vi "1_test_1.vi"() -> ()   [LabVIEW 2020]
uses:
  <vilib>/Utility/file.llb/Write Delimited Spreadsheet (DBL).vi
  <vilib>/regexp/Match Regular Expression.xnode
panel:
  out "类型":string
  out "倒数第二步骤 2":string
  out "倒数第三步骤":string
  out "文档名称":string
  out "当前路径文件为：":string
  in  "数字":dbl
  in  "字符串 3":string
  in  "模板初始文档地址":string
  out "当前文件读取为：":string
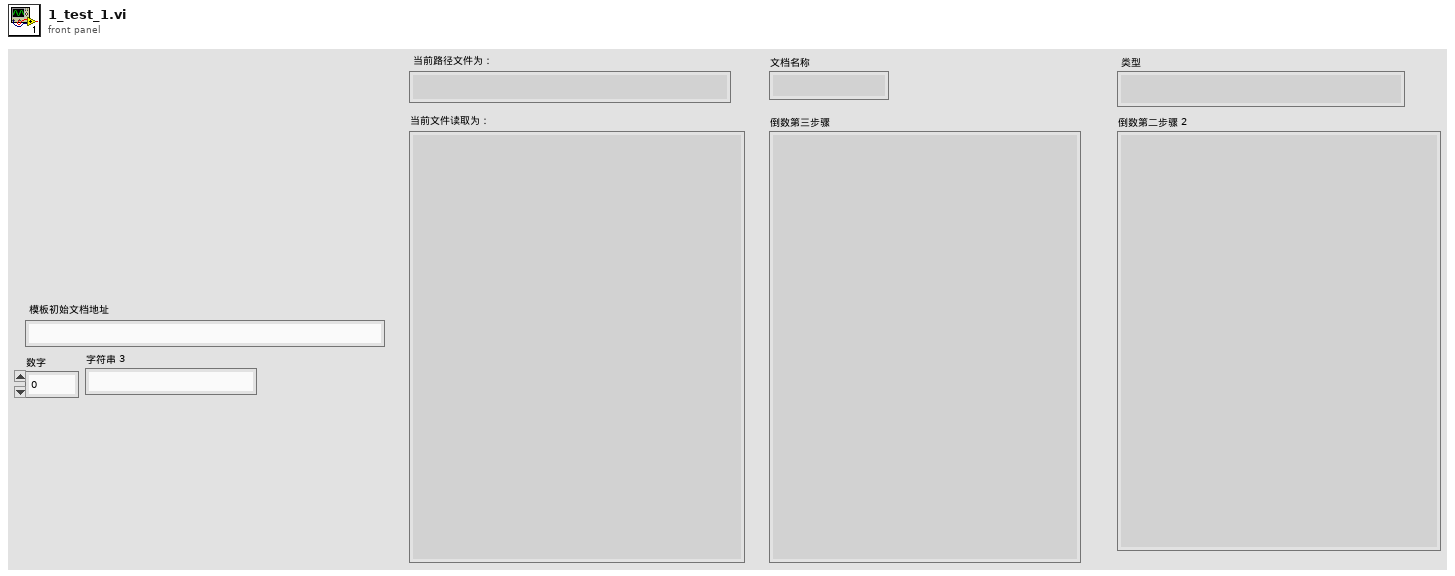
[diagram p1: front panel]
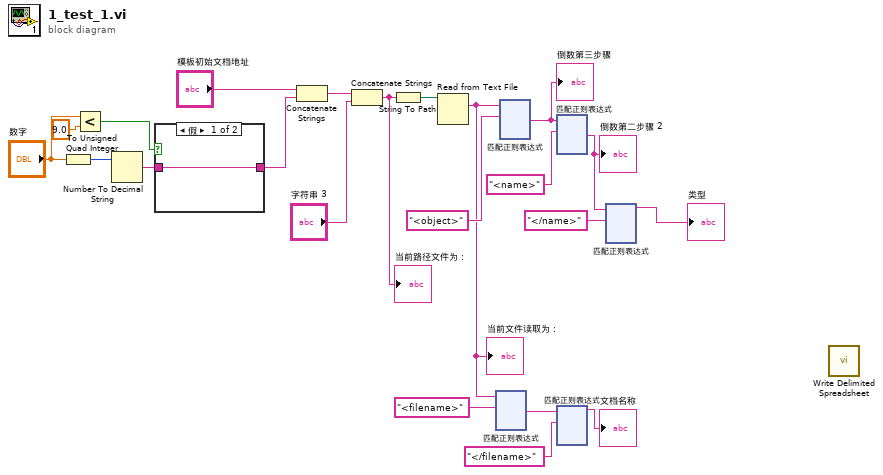
[diagram p0: block diagram]
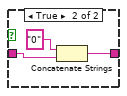
[diagram p2: hidden frame]
diagram:
  n1 = To Unsigned Quad Integer(1:"数字") -> (0:w19:u64)
  n2 = Less?(x="数字", y=9.0) -> (x < y?=w16:bool)
  n3 = Number To Decimal String(number=w19) -> (decimal integer string=w14:string)  [unwired: 1 in]
  n4 = case shown="假" w16 {
    tunnel: w14 -> [w23 w25]
    tunnel: [w23 w24] -> w13
    frame False {
    }
    frame True {
      n5 = Concatenate Strings("0" ("字符串"), w25) -> (w24:string)
    }
  }
  n6 = Concatenate Strings("模板初始文档地址", w13) -> (w20:string)
  n7 = Concatenate Strings(w20, "字符串 3") -> (w18:string)
  "当前路径文件为：" <- w18
  n8 = String To Path(string=w18) -> (path=w12:path)
  n9 = Read from Text File(file (use dialog)=w12) -> (text=w5:string)  [unwired: 3 in, 3 out]
  "当前文件读取为：" <- w5
  n10 = xnode "匹配正则表达式"("输入字符串"=w5, "正则表达式"="<filename>") -> ("匹配之后"=w10:string)  [unwired: 4 in, 4 out]
  n11 = xnode "匹配正则表达式"("输入字符串"=w5, "正则表达式"="<object>") -> ("匹配之后"=w4:string)  [unwired: 4 in, 4 out]
  "倒数第三步骤" <- w4
  n12 = xnode "匹配正则表达式"("输入字符串"=w4, "正则表达式"="<name>") -> ("匹配之后"=w3:string)  [unwired: 4 in, 4 out]
  "倒数第二步骤 2" <- w3
  n13 = xnode "匹配正则表达式"("输入字符串"=w10, "正则表达式"="</filename>") -> ("匹配之前"=→"文档名称":string)  [unwired: 4 in, 4 out]
  n14 = xnode "匹配正则表达式"("输入字符串"=w3, "正则表达式"="</name>") -> ("匹配之前"=→"类型":string)  [unwired: 4 in, 4 out]
  n15 = call-poly <vilib>:"Write Delimited Spreadsheet.vi"() -> ()  [unwired: 14 in, 2 out]
